vi "Add a Compact PDO.vi"(6 "RX?":bool, 7 "Arr Refnum":refnum<vi>, 8 "error in (no error)":errorcluster, 9 "Index of Compact PDO":u16[](array[numeric]), 10 "Count of Sub Items":i32, 11 "Start":u16) -> (0 "error out":errorcluster)   [LabVIEW 2021, in "CANOpen Addon System Explorer.lvlib"]
uses:
  CANOpen Addon System Explorer.lvlib
  control/OD Entry.ctl
  control/Object Type.ctl
  control/Data Type.ctl
  control/Access Type.ctl
  control/OD Cateory.ctl
panel:
  in  "TPDO":T1[](array[typedef])=[{"index"=0, "sub-index"=0, "Level"=0, "ObjectType"=9, "DataType"=0, "ParameterName"="TPDO communication parameter", "LowLimit"="", "HighLimit"="", "AccessType"=0, "DefaultValue"="", "PDOMapping"=FALSE, "SubNumber"=0, "ObjFlags"=0, "Category"=enum."Optional"}, {"index"=0, "sub-index"=0, "Level"=1, "ObjectType"=7, "DataType"=5, "ParameterName"="highest sub-index supported", "LowLimit"="0x2", "HighLimit"="0x6", "AccessType"=1, "DefaultValue"="", "PDOMapping"=FALSE, "SubNumber"=0, "ObjFlags"=0, "Category"=enum."Mandatory"}, {"index"=0, "sub-index"=1, "Level"=1, "ObjectType"=7, "DataType"=7, "ParameterName"="COB-ID used by TPDO", "LowLimit"="", "HighLimit"="", "AccessType"=3, "DefaultValue"="", "PDOMapping"=FALSE, "SubNumber"=0, "ObjFlags"=0, "Category"=enum."Mandatory"}, {"index"=0, "sub-index"=2, "Level"=1, "ObjectType"=7, "DataType"=5, "ParameterName"="transmission type", "LowLimit"="", "HighLimit"="", "AccessType"=3, "DefaultValue"="", "PDOMapping"=FALSE, "SubNumber"=0, "ObjFlags"=0, "Category"=enum."Mandatory"}, {"index"=0, "sub-index"=3, "Level"=1, "ObjectType"=7, "DataType"=6, "ParameterName"="inhibit time", "LowLimit"="", "HighLimit"="", "AccessType"=3, "DefaultValue"="", "PDOMapping"=FALSE, "SubNumber"=0, "ObjFlags"=0, "Category"=enum."Mandatory"}, {"index"=0, "sub-index"=4, "Level"=1, "ObjectType"=7, "DataType"=5, "ParameterName"="compatibility entry", "LowLimit"="", "HighLimit"="", "AccessType"=3, "DefaultValue"="", "PDOMapping"=FALSE, "SubNumber"=0, "ObjFlags"=0, "Category"=enum."Mandatory"}, {"index"=0, "sub-index"=5, "Level"=1, "ObjectType"=7, "DataType"=6, "ParameterName"="event-timer", "LowLimit"="", "HighLimit"="", "AccessType"=3, "DefaultValue"="", "PDOMapping"=FALSE, "SubNumber"=0, "ObjFlags"=0, "Category"=enum."Mandatory"}, {"index"=0, "sub-index"=6, "Level"=1, "ObjectType"=7, "DataType"=5, "ParameterName"="SYNC start value", "LowLimit"="", "HighLimit"="", "AccessType"=3, "DefaultValue"="", "PDOMapping"=FALSE, "SubNumber"=0, "ObjFlags"=0, "Category"=enum."Mandatory"}] {"SubNumber" format="%x"; "AccessType" items=["", "ro", "wo", "rw", "const", "rwr", "rww"]; "DataType" items=[""=0, "BOOLEAN"=1, "INTEGER8"=2, "INTEGER16"=3, "INTEGER32"=4, "UNSIGNED8"=5, "UNSIGNED16"=6, "UNSIGNED32"=7, "REAL32"=8, "VISIBLE_STRING"=9, "OCTET_STRING"=10, "UNICODE_STRING"=11, "TIME_OF_DAY"=12, "TIME_DIFFERENCE"=13, "DOMAIN"=15, "INTEGER24"=16, "REAL64"=17, "INTEGER40"=18, "INTEGER48"=19, "INTEGER56"=20, "INTEGER64"=21, "UNSIGNED24"=22, "UNSIGNED40"=24, "UNSIGNED48"=25, "UNSIGNED56"=26, "UNSIGNED64"=27]; "ObjectType" items=[""=10, "NULL"=0, "DOMAIN"=2, "DEFTYPE"=5, "DEFSTRUCT"=6, "VAR"=7, "ARRAY"=8, "RECORD"=9]; "sub-index" format="%x"; "index" format="%x"}
  in  "RPDO":T1[](array[typedef])=[{"index"=0, "sub-index"=0, "Level"=0, "ObjectType"=9, "DataType"=0, "ParameterName"="RPDO communication parameter", "LowLimit"="", "HighLimit"="", "AccessType"=0, "DefaultValue"="", "PDOMapping"=FALSE, "SubNumber"=0, "ObjFlags"=0, "Category"=enum."Optional"}, {"index"=0, "sub-index"=0, "Level"=1, "ObjectType"=7, "DataType"=5, "ParameterName"="highest sub-index supported", "LowLimit"="0x2", "HighLimit"="0x6", "AccessType"=1, "DefaultValue"="", "PDOMapping"=FALSE, "SubNumber"=0, "ObjFlags"=0, "Category"=enum."Mandatory"}, {"index"=0, "sub-index"=1, "Level"=1, "ObjectType"=7, "DataType"=7, "ParameterName"="COB-ID used by RPDO", "LowLimit"="", "HighLimit"="", "AccessType"=3, "DefaultValue"="", "PDOMapping"=FALSE, "SubNumber"=0, "ObjFlags"=0, "Category"=enum."Mandatory"}, {"index"=0, "sub-index"=2, "Level"=1, "ObjectType"=7, "DataType"=5, "ParameterName"="transmission type", "LowLimit"="", "HighLimit"="", "AccessType"=3, "DefaultValue"="", "PDOMapping"=FALSE, "SubNumber"=0, "ObjFlags"=0, "Category"=enum."Mandatory"}, {"index"=0, "sub-index"=3, "Level"=1, "ObjectType"=7, "DataType"=6, "ParameterName"="inhibit time", "LowLimit"="", "HighLimit"="", "AccessType"=3, "DefaultValue"="", "PDOMapping"=FALSE, "SubNumber"=0, "ObjFlags"=0, "Category"=enum."Mandatory"}, {"index"=0, "sub-index"=4, "Level"=1, "ObjectType"=7, "DataType"=5, "ParameterName"="compatibility entry", "LowLimit"="", "HighLimit"="", "AccessType"=3, "DefaultValue"="", "PDOMapping"=FALSE, "SubNumber"=0, "ObjFlags"=0, "Category"=enum."Mandatory"}, {"index"=0, "sub-index"=5, "Level"=1, "ObjectType"=7, "DataType"=6, "ParameterName"="event-timer", "LowLimit"="", "HighLimit"="", "AccessType"=3, "DefaultValue"="", "PDOMapping"=FALSE, "SubNumber"=0, "ObjFlags"=0, "Category"=enum."Mandatory"}, {"index"=0, "sub-index"=6, "Level"=1, "ObjectType"=7, "DataType"=5, "ParameterName"="SYNC start value", "LowLimit"="", "HighLimit"="", "AccessType"=3, "DefaultValue"="", "PDOMapping"=FALSE, "SubNumber"=0, "ObjFlags"=0, "Category"=enum.""}] {"SubNumber" format="%x"; "AccessType" items=["", "ro", "wo", "rw", "const", "rwr", "rww"]; "DataType" items=[""=0, "BOOLEAN"=1, "INTEGER8"=2, "INTEGER16"=3, "INTEGER32"=4, "UNSIGNED8"=5, "UNSIGNED16"=6, "UNSIGNED32"=7, "REAL32"=8, "VISIBLE_STRING"=9, "OCTET_STRING"=10, "UNICODE_STRING"=11, "TIME_OF_DAY"=12, "TIME_DIFFERENCE"=13, "DOMAIN"=15, "INTEGER24"=16, "REAL64"=17, "INTEGER40"=18, "INTEGER48"=19, "INTEGER56"=20, "INTEGER64"=21, "UNSIGNED24"=22, "UNSIGNED40"=24, "UNSIGNED48"=25, "UNSIGNED56"=26, "UNSIGNED64"=27]; "ObjectType" items=[""=10, "NULL"=0, "DOMAIN"=2, "DEFTYPE"=5, "DEFSTRUCT"=6, "VAR"=7, "ARRAY"=8, "RECORD"=9]; "sub-index" format="%x"; "index" format="%x"}
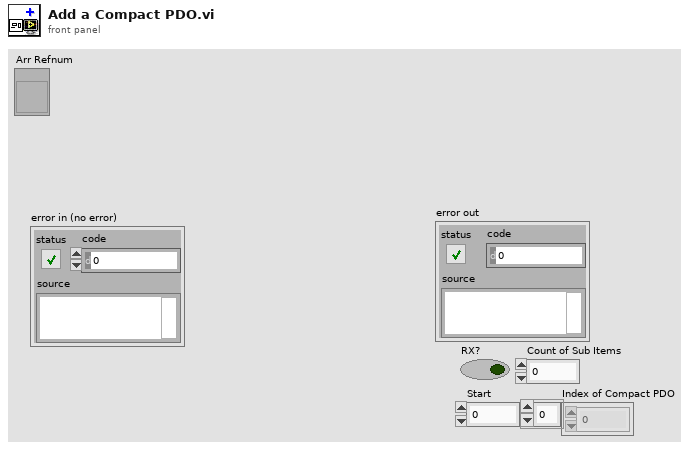
[diagram p1: front panel]
types:
  T1 = typedef "CANOpen Addon System Explorer.lvlib/OD Entry.ctl" = cluster{"index":u16, "sub-index":u8, "Level":u8, "ObjectType":T2, "DataType":T3, "ParameterName":string, "LowLimit":string, "HighLimit":string, "AccessType":T4, "DefaultValue":string, "PDOMapping":bool, "SubNumber":u8, "ObjFlags":u32, "Category":T5}
  T2 = typedef "CANOpen Addon System Explorer.lvlib/Object Type.ctl" = u16
  T3 = typedef "CANOpen Addon System Explorer.lvlib/Data Type.ctl" = u16
  T4 = typedef "CANOpen Addon System Explorer.lvlib/Access Type.ctl" = u16
  T5 = typedef "CANOpen Addon System Explorer.lvlib/OD Cateory.ctl" = enum16{"Mandatory", "Optional", "Manufacturer", ""}
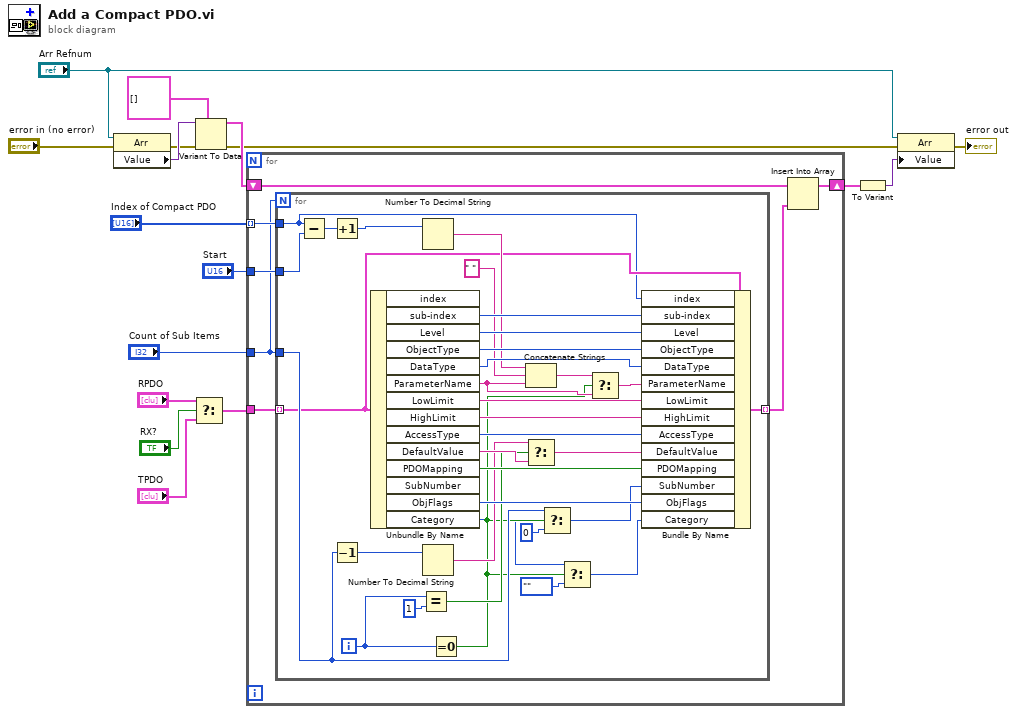
[diagram p0: block diagram]
diagram:
  n1 = property class="Arr"(reference="Arr Refnum", error in="error in (no error)") -> (error out=w13:errorcluster, "Value"=w14:variant)  [unwired: 1 out]
  n2 = Select(t="RPDO", s="RX?", f="TPDO") -> (s? t:f=w8:T1[])
  n3 = Variant To Data(error in=w13, type=T1[] [], Variant=w14) -> (data=w7:T1[], error out=w5:errorcluster)
  n4 = for {
    tunnel: "Index of Compact PDO" -> [w24] mode=indexing
    tunnel: "Start" -> [w23]
    tunnel: w8 -> [w22]
    tunnel: "Count of Sub Items" -> [w18]
    shift-right: [w19] -> w6
    shift-left: w7 -> [w21]
    n5 = for {
      N: w18 -> [_]
      tunnel: [w49] -> w20 mode=indexing
      tunnel: w18 -> [w33]
      tunnel: w24 -> [w29]
      tunnel: w23 -> [w31]
      tunnel: w22 -> [w30] mode=indexing
      i -> [w38]
      n6 = Subtract(x=w29, y=w31) -> (x-y=w41:u16)
      n7 = Increment(x=w41) -> (x+1=w32:u16)
      n8 = Decrement(x=w33) -> (x-1=w34:i32)
      n9 = Unbundle By Name(w30) -> ("sub-index"=w50:u8, "Level"=w51:u8, "ObjectType"=w52:T2, "DataType"=w53:T3, "ParameterName"=w43:string, "LowLimit"=w58:string, "HighLimit"=w57:string, "AccessType"=w56:T4, "DefaultValue"=w40:string, "PDOMapping"=w55:bool, "ObjFlags"=w54:u32, "Category"=w27:T5)  [unwired: 2 out]
      n10 = Equal?(x=w38, y=1) -> (x = y?=w36:bool)
      n11 = Number To Decimal String(number=w32) -> (decimal integer string=w44:string)  [unwired: 1 in]
      n12 = Number To Decimal String(number=w34) -> (decimal integer string=w35:string)  [unwired: 1 in]
      n13 = Equal To 0?(x=w38) -> (x = 0?=w28:bool)
      n14 = Concatenate Strings(w44, " " ("string"), w43) -> (w46:string)
      n15 = Select(t=w35, s=w36, f=w40) -> (s? t:f=w39:string)
      n16 = Select(t=w33, s=w28, f=u8 0) -> (s? t:f=w48:i32)
      n17 = Select(t=w27, s=w28, f=OD_Cateory."") -> (s? t:f=w25:T5)
      n18 = Select(t=w46, s=w28, f=w43) -> (s? t:f=w42:string)
      n19 = Bundle By Name(cluster=w30, "index"=w29, "sub-index"=w50, "Level"=w51, "ObjectType"=w52, "DataType"=w53, "ParameterName"=w42, "LowLimit"=w58, "HighLimit"=w57, "AccessType"=w56, "DefaultValue"=w39, "PDOMapping"=w55, "SubNumber"=w48, "ObjFlags"=w54, "Category"=w25) -> (w49:T1)
    }
    n20 = Insert Into Array(array=w21, new element=w20) -> (w19:T1[])  [unwired: 1 in]
  }
  n21 = To Variant(anything=w6) -> (Variant=w10:variant)
  n22 = property class="Arr"(reference="Arr Refnum", error in=w5, "Value"=w10) -> (error out=→"error out":errorcluster)  [unwired: 1 out]
